vi "Open.vi"(8 "error in (no error)":errorcluster, 10 "Session In":T1="S1019101", 11 "CameraLan in":refnum<class "CameraLan.lvclass">) -> (0 "error out":errorcluster, 3 "CameraLan out":refnum<class "CameraLan.lvclass">)   [LabVIEW 2013, in "CameraLan.lvclass"]
uses:
  CameraLan.lvclass
  <vilib>/userdefined/High Color/IMAQdx.ctl
  CameraLan.lvclass/CameraLan.ctl
  <vilib>/vision/driver/NI_Vision_Acquisition_Software.lvlib
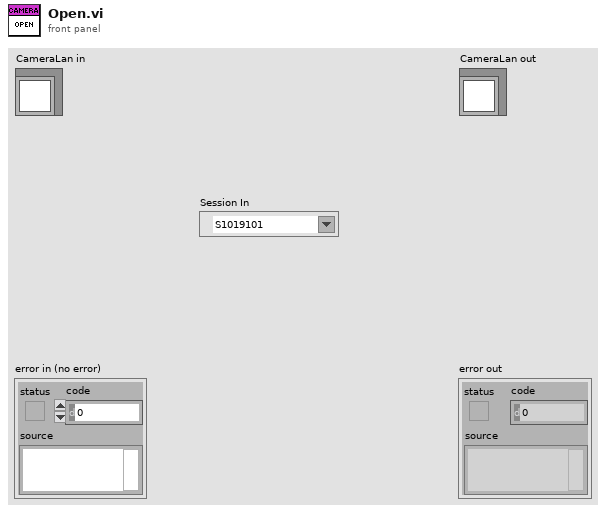
[diagram p1: front panel]
types:
  T1 = typedef "IMAQdx.ctl" = refnum<k21>
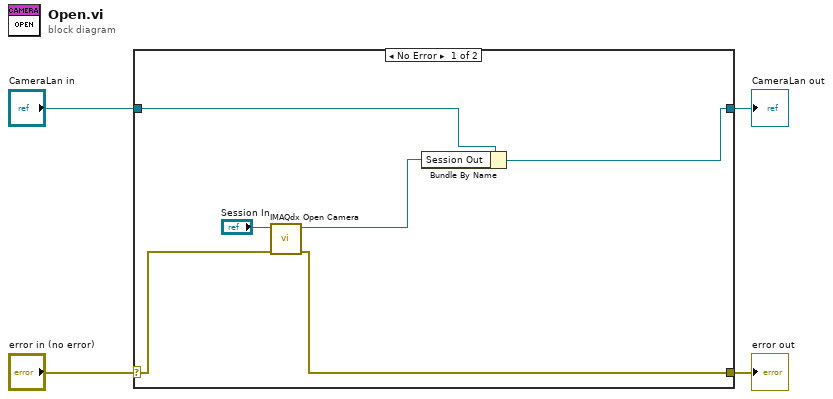
[diagram p0: block diagram]
diagram:
  n1 = case shown="No Error" "error in (no error)" {
    selector: "error in (no error)" -> [w6 w12]
    tunnel: [w5 w12] -> w3
    tunnel: [w9 w11] -> w1
    tunnel: "CameraLan in" -> [w10 w11]
    frame No Error {
      n2 = call <vilib>:"IMAQdx Open Camera.vi"("error in"=w6, "Session In"="Session In") -> ("error out"=w5:errorcluster, "Session Out"=w8:T1)  [unwired: 1 in, 7 out]
      n3 = Bundle By Name(cluster=w10, "Session Out"=w8) -> (w9:refnum<class "CameraLan.lvclass">)
    }
    frame Error {
    }
  }
  "error out" <- w3
  "CameraLan out" <- w1
